vi "sc_absXYZ.vi"(6 "abs Z (steps)":i32, 8 "error in (no error)":errorcluster, 9 "abs Y (steps)":i32, 10 "abs X (steps)":i32, 11 "VISA handle":refnum<visa-resource-name>) -> (0 "error out":errorcluster, 2 "argument integer string":string, 3 "Dup. VISA handle":refnum<visa-resource-name>)   [LabVIEW 2019]
uses:
  controls/scientifica_commands.ctl
panel:
  out "Response":string
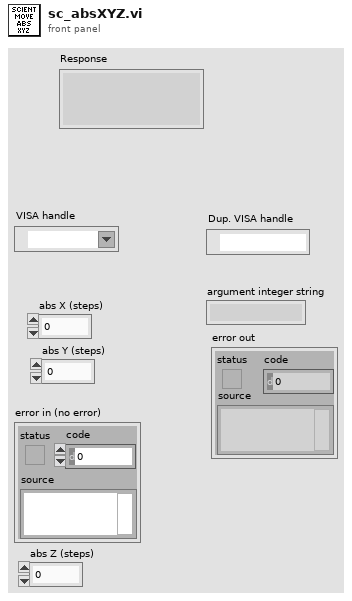
[diagram p1: front panel]
types:
  T1 = typedef "scientifica_commands.ctl" = enum16{"ANGLE", "INSET", "FIRST", "ZERO", "Pz", "P", "absz", "ACC", "TOP", "STOP", "rel", "relz", "abs", "IN", "vj", "APROACH", "OBJS", "OBJU", "OUT", "OBJ", "OBJL", "SET", "OBJD", "STEP", "SETSTEP", "S", "UUX", "UUY", "UUZ"}
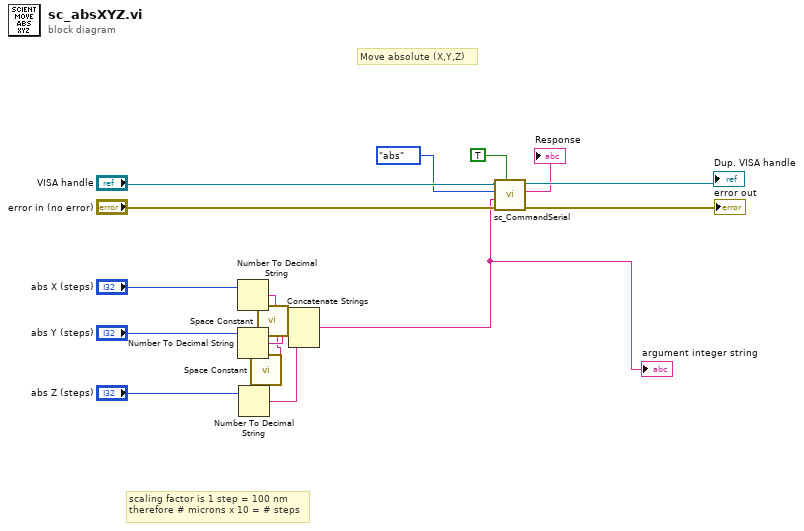
[diagram p0: block diagram]
diagram:
  # "scaling factor is 1 step = 100 nm\ntherefore # microns x 10 = # steps"
  # "Move absolute (X,Y,Z)"
  n1 = Number To Decimal String(number="abs X (steps)") -> (decimal integer string=w10:string)  [unwired: 1 in]
  n2 = Number To Decimal String(number="abs Y (steps)") -> (decimal integer string=w8:string)  [unwired: 1 in]
  n3 = Number To Decimal String(number="abs Z (steps)") -> (decimal integer string=w2:string)  [unwired: 1 in]
  n4 = call <vilib>:"Space Constant.vi"() -> ("String"=w4:string)
  n5 = call <vilib>:"Space Constant.vi"() -> ("String"=w9:string)
  n6 = Concatenate Strings(w10, w9, w8, w4, w2) -> (w7:string)
  "argument integer string" <- w7
  n7 = call "sc_CommandSerial.vi"("Query?"=TRUE, "error in (no error)"="error in (no error)", "argument"=w7, "Scientifica commands"=scientifica_commands."abs", "VISA handle"="VISA handle") -> ("error out"=→"error out":errorcluster, "Response"=→"Response":string, "Dup. VISA handle"=→"Dup. VISA handle":refnum<visa-resource-name>)  [unwired: 3 in, 1 out]
